vi "Calibrering.vi"(10 "Array":dbl[](array[numeric]), 11 "Cal(F.L)":dbl[](array[numeric])) -> (2 "Kg":dbl[](array[numeric]), 3 "sum":dbl)   [LabVIEW 2019]
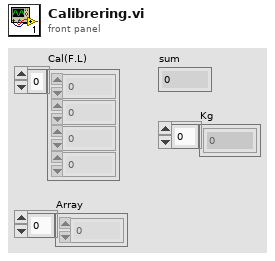
[diagram p1: front panel]
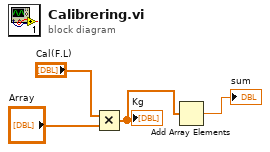
[diagram p0: block diagram]
diagram:
  n1 = Multiply(x="Cal(F.L)", y="Array") -> (x*y=w3:dbl[])
  "Kg" <- w3
  n2 = Add Array Elements(numeric array=w3) -> (sum=→"sum":dbl)
